vi "digital_output_all_config.vi"() -> ()   [LabVIEW 2024]
uses:
  <vilib>/DAQmx/write.llb/DAQmx Write (Digital 1D Bool 1Chan 1Samp).vi
  <vilib>/DAQmx/create/channels.llb/DAQmx Create Channel (DO-Digital Output).vi
  <vilib>/DAQmx/miscellaneous.llb/DAQmx Fill In Error Info.vi
panel:
  in  "data":bool[](array[boolean])
  out "error out":errorcluster
  in  "lines":tag
  in  "stop":bool
  # "Se leen las entradas digitales utilizando una \"task\"\nconfigurada en NI MAX con el nombre \"read_collector\""
  # "DAQ utilizado NI USB 6009"
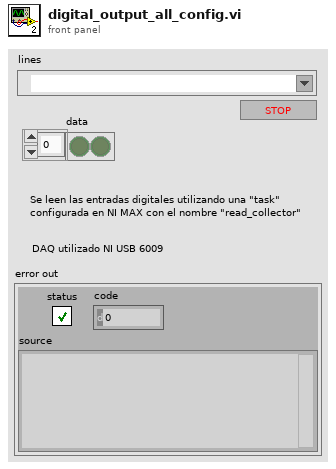
[diagram p1: front panel]
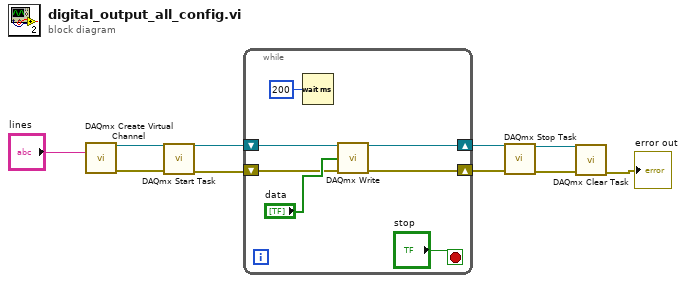
[diagram p0: block diagram]
diagram:
  n1 = call-poly <vilib>:"DAQmx Create Virtual Channel.vi"("lines"="lines") -> ("task out"=w5:refnum<k21>, "error out"=w4:errorcluster)  [unwired: 13 in]
  n2 = call <vilib>:"DAQmx Start Task.vi"("task/channels in"=w5, "error in"=w4) -> ("task out"=w3:refnum<k21>, "error out"=w2:errorcluster)  [unwired: 12 in]
  n3 = while {
    shift-right: [w12] -> w10
    shift-left: w3 -> [w14]
    shift-right: [w11] -> w9
    shift-left: w2 -> [w13]
    stop <- "stop" stop-if-true
    n4 = Wait (ms)(milliseconds to wait=u32 200) -> ()  [unwired: 1 out]
    n5 = call-poly <vilib>:"DAQmx Write.vi"("task/channels in"=w14, "data"="data", "error in"=w13) -> ("task out"=w12:refnum<k21>, "error out"=w11:errorcluster)  [unwired: 10 in, 1 out]
  }
  n6 = call <vilib>:"DAQmx Stop Task.vi"("task/channels in"=w10, "error in"=w9) -> ("task out"=w8:refnum<k21>, "error out"=w7:errorcluster)  [unwired: 12 in]
  n7 = call <vilib>:"DAQmx Clear Task.vi"("task in"=w8, "error in"=w7) -> ("error out"=→"error out":errorcluster)  [unwired: 13 in]
